vi "Settings Register.vi"(3 "error in (no error)":errorcluster, 4 "Set Settings":T1={"Pixel clock"=20, "Frame rate"=30.0, "Exposure time"=33.21525, "Master Gain"=0, "Red Gain"=0, "Green Gain"=0, "Blue Gain"=0, "Auto Gain"=FALSE, "White-balance"=FALSE, "Color Correction"=FALSE} {"Blue Gain" min=0 max=100 step=1 scale=0.0..100.0; "Green Gain" min=0 max=100 step=1 scale=0.0..100.0; "Red Gain" min=0 max=100 step=1 scale=0.0..100.0; "Master Gain" min=0 max=100 step=1 scale=0.0..100.0; "Exposure time" min=0.06675 max=99.92475 step=0.06675 scale=0.06675..99.92475 scale format="%#.3g"; "Frame rate" min=4.876716604244694 max=13.962044182888818 step=6.675e-05 scale=13.962044182888818..15.3582486011777 scale format="%^#_3g"; "Pixel clock" min=5 max=43 step=1 scale=5.0..43.0}, 5 "Function":enum16{"Get", "Set", "Start", "Stop"}(ring)) -> (0 "error out":errorcluster, 1 "Get Settings":T1={"Pixel clock"=20, "Frame rate"=30.0, "Exposure time"=33.21525, "Master Gain"=0, "Red Gain"=0, "Green Gain"=0, "Blue Gain"=0, "Auto Gain"=FALSE, "White-balance"=FALSE, "Color Correction"=FALSE} {"Blue Gain" min=0 max=100 step=1 scale=0.0..100.0; "Green Gain" min=0 max=100 step=1 scale=0.0..100.0; "Red Gain" min=0 max=100 step=1 scale=0.0..100.0; "Master Gain" min=0 max=100 step=1 scale=0.0..100.0; "Exposure time" min=0.06675 max=99.92475 step=0.06675 scale=0.06675..99.92475 scale format="%#.3g"; "Frame rate" min=4.876716604244694 max=13.962044182888818 step=6.675e-05 scale=13.962044182888818..15.3582486011777 scale format="%^#_3g"; "Pixel clock" min=5 max=43 step=1 scale=5.0..43.0}, 2 "Acquire?":bool)   [LabVIEW 2014]
uses:
  Camera Settings.ctl
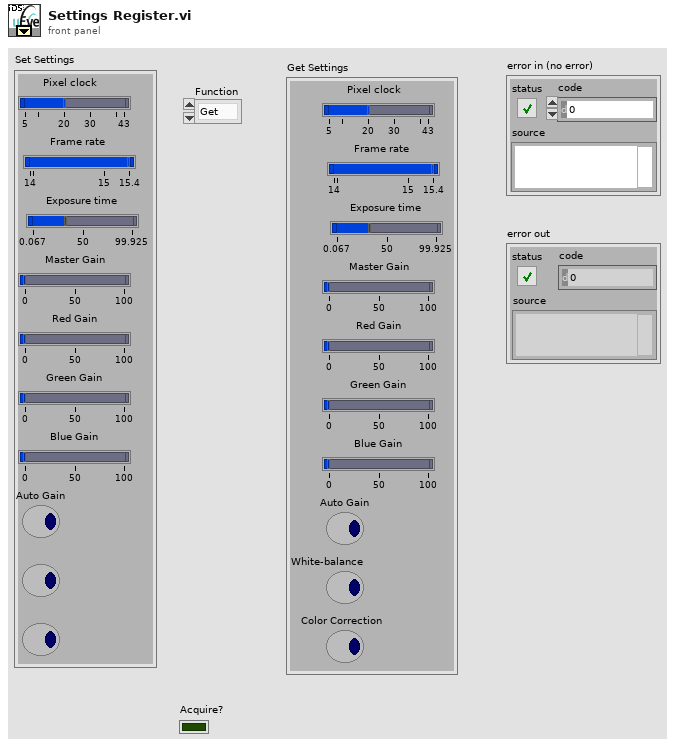
[diagram p1: front panel]
types:
  T1 = typedef "Camera Settings.ctl" = cluster{"Pixel clock":i32, "Frame rate":dbl, "Exposure time":dbl, "Master Gain":i32, "Red Gain":i32, "Green Gain":i32, "Blue Gain":i32, "Auto Gain":bool, "White-balance":bool, "Color Correction":bool}
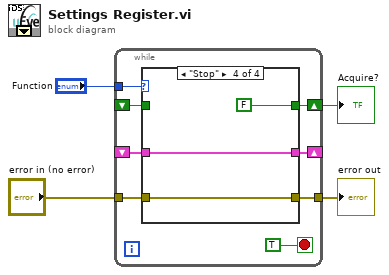
[diagram p0: block diagram]
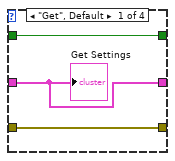
[diagram p2: hidden frame]
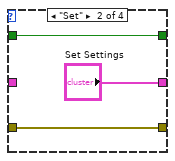
[diagram p3: hidden frame]
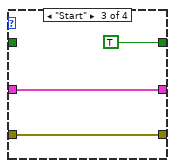
[diagram p4: hidden frame]
diagram:
  n1 = while {
    tunnel: "Function" -> [w12]
    shift-right: [w10] -> _
    shift-left: _ -> [w11]
    tunnel: [w8] -> w3
    tunnel: "error in (no error)" -> [w7]
    shift-right: [w5] -> w1
    shift-left: _ -> [w6]
    stop <- TRUE stop-if-true
    n2 = case shown="\"Stop\"" w12 {
      tunnel: w11 -> [w15 _ w20 w23]
      tunnel: [w15 "Set Settings" w20 w23] -> w10
      tunnel: [w14 w17 w21 w24] -> w8
      tunnel: w7 -> [w14 w17 w21 w24]
      tunnel: w6 -> [w13 w16 _ _]
      tunnel: [w13 w16 TRUE ("Acquire? 2") FALSE ("Acquire? 2")] -> w5
      frame "Get", Default {
        "Get Settings" <- w15
      }
      frame "Set" {
      }
      frame "Start" {
      }
      frame "Stop" {
      }
    }
  }
  "error out" <- w3
  "Acquire?" <- w1
